vi "Create HELLO msg (JSON).vi"(6 "aututhextras":string, 8 "error in (no error)":errorcluster, 9 "Authmethods":string[](array[string]), 10 "Auth ID":string, 11 "Realm":string) -> (0 "error out":errorcluster, 3 "WAMP message":string)   [LabVIEW 2020, in "wamplv.lvlib" / "WAMP Client.lvclass"]
uses:
  WAMP Client.lvclass
  Private/TypeDefs/WAMP Message Codes.ctl
  3e6dd2ed-6f17-45bb-8da1-37bc315f6a7e.vi
  <vilib>/JDP Science/JSONtext/Variant to JSON Text.vi
  <vilib>/JDP Science/JSONtext/LVClass Serializer/JSONtext LVClass Serializer.lvclass
  WAMP Client.lvclass/WAMP Client.ctl
  wamplv.lvlib
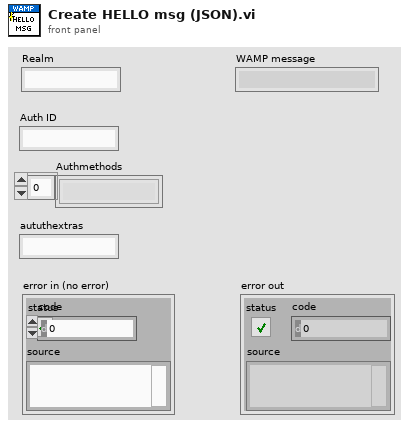
[diagram p1: front panel]
types:
  T1 = typedef "wamplv.lvlib/WAMP Message Codes.ctl" = u16
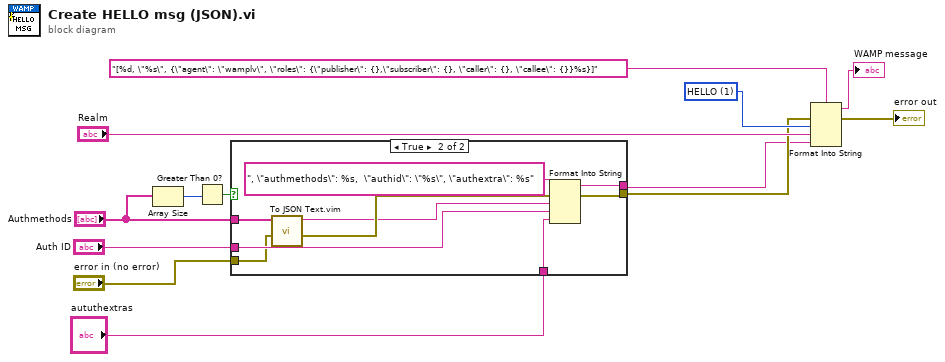
[diagram p0: block diagram]
diagram:
  w9 = T1 1 items=["HELLO"=1, "WELCOME"=2, "ABORT"=3, "GOODBYE"=6, "ERROR"=8, "PUBLISH"=16, "PUBLISHED"=17, "SUBSCRIBE"=32, "SUBSCRIBED"=33, "UNSUBSCRIBE"=34, "UNSUBSCRIBED"=35, "EVENT"=36, "CALL"=48, "RESULT"=59, "REGISTER"=64, "REGISTERED"=65, "UNREGISTER"=66, "UNREGISTERED"=67, "INVOCATION"=68, "YIELD"=70] ("Message Codes")
  n1 = Array Size(array="Authmethods") -> (size(s)=w8:i32)
  n2 = Greater Than 0?(x=w8) -> (x > 0?=w7:bool)
  n3 = case shown="True" w7 {
    tunnel: "Authmethods" -> [_ w19]
    tunnel: "error in (no error)" -> [w14 w18]
    tunnel: "Auth ID" -> [_ w22]
    tunnel: [w14 w21] -> w3
    tunnel: [_ w20] -> w2
    tunnel: "aututhextras" -> [_ w15]
    frame False {
    }
    frame True {
      n4 = call "To JSON Text.vim"("error in (no error)"=w18, "Anything"=w19) -> ("error out"=w17:errorcluster, "<JSON>"=w16:string)  [unwired: 8 in]
      n5 = Format Into String(format string=", \"authmethods\": %s,  \"authid\": \"%s\", \"authextra\": %s", error in=w17, w16, w22, w15) -> (resulting string=w20:string, error out=w21:errorcluster)  [unwired: 1 in]
    }
  }
  n6 = Format Into String(format string="[%d, \"%s\", {\"agent\": \"wamplv\", \"roles\": {\"publisher\": {},\"subscriber\": {}, \"caller\": {}, \"callee\": {}}%s}]", error in=w3, w9, "Realm", w2) -> (resulting string=→"WAMP message":string, error out=→"error out":errorcluster)  [unwired: 1 in]
